vi "CANOpen_Create PDO and Channels.vi"(7 "Type":T1, 8 "error in (no error)":errorcluster, 9 "Cancelled?":bool, 10 "PDO Settings":T3={"Parameters"=[], "PDO Channel"=1, "Start Index"=0, "Length"=0} {"PDO Channel" items=["PDO 1", "PDO 2", "PDO 3", "PDO 4"]; "Parameters"."Bit Offset" max=8 step=1; "Parameters"."Byte Offset" max=8 step=1}, 11 "Item Ref out":T2 format="%.0x") -> (0 "error out":errorcluster, 2 "New PDO":T2=18446744073709551615 format="%.0x")   [LabVIEW 2013]
uses:
  <vilib>/NI Veristand/Custom Device API/Custom Device Item Ref.ctl
  Shared Code/CANOpen_PDO Settings.ctl
  Shared Code/CANOpen_PDO Parameter Settings.ctl
  Shared Code/CANOpen_PDO Data Type.ctl
  CANopen Byte Order.ctl
  CANOpen_PDO Type.ctl
  <vilib>/NI Veristand/Custom Device API/Custom Device Channel.ctl
  <vilib>/NI Veristand/Custom Device API/Custom Device Channel Type.ctl
  Shared Code/CANOpen Addon GUID Lookup Global.vi
  CANOpen Addon Custom Device.lvlib
  <vilib>/NI Veristand/Custom Device API/Custom Device API.lvlib
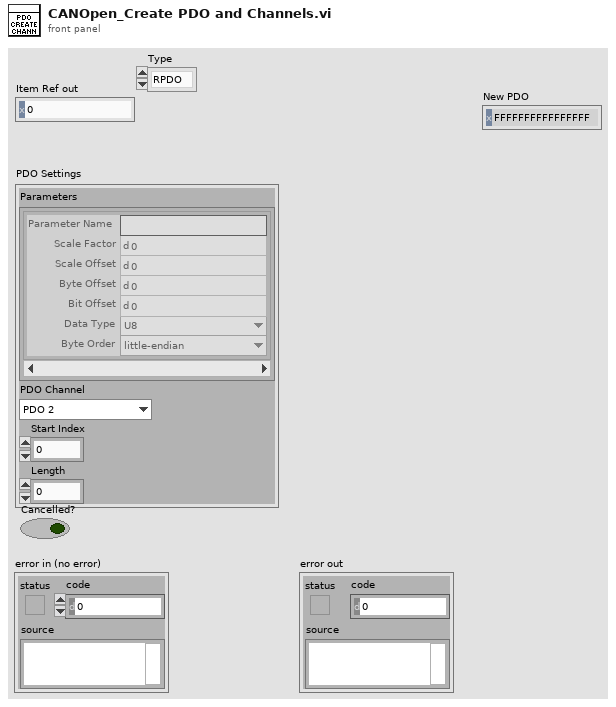
[diagram p1: front panel]
types:
  T1 = typedef "CANOpen_PDO Type.ctl" = enum16{"RPDO", "TPDO"}
  T2 = typedef "Custom Device API.lvlib/Custom Device Item Ref.ctl" = u64
  T3 = typedef "CANOpen Addon Custom Device.lvlib/CANOpen_PDO Settings.ctl" = cluster{"Parameters":T4[], "PDO Channel":u8, "Start Index":u32, "Length":u32}
  T4 = typedef "CANOpen Addon Custom Device.lvlib/CANOpen_PDO Parameter Settings.ctl" = cluster{"Parameter Name":string, "Scale Factor":dbl, "Scale Offset":dbl, "Byte Offset":u8, "Bit Offset":u8, "Data Type":T5, "Byte Order":T6}
  T5 = typedef "CANOpen Addon Custom Device.lvlib/CANOpen_PDO Data Type.ctl" = enum16{"U8", "U16", "U32", "I8", "I16", "I32", "Single", "Double", "Boolean"}
  T6 = typedef "CANOpen Addon Custom Device.lvlib/CANopen Byte Order.ctl" = enum16{"big-endian network order", "little-endian"}
  T7 = typedef "Custom Device API.lvlib/Custom Device Channel.ctl" = cluster{"Type":T8, "Units":string, "Default Value":dbl, "Faultable":bool, "Scalable":bool}
  T8 = typedef "Custom Device API.lvlib/Custom Device Channel Type.ctl" = enum16{"Input", "Output"}
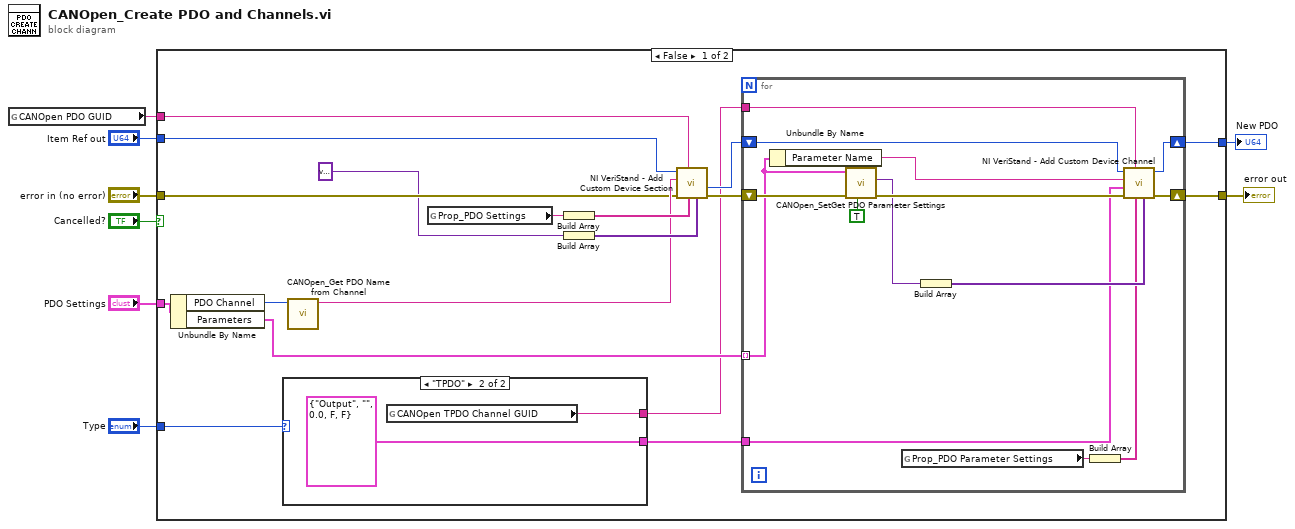
[diagram p0: block diagram]
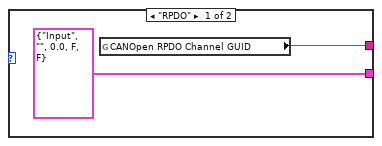
[diagram p2: hidden frame]
diagram:
  n1 = global read "CANOpen Addon GUID Lookup Global.vi" "CANOpen PDO GUID"() -> (w7:string)
  n2 = case shown="False" "Cancelled?" {
    tunnel: w7 -> [w26 _]
    tunnel: [w17 w45] -> w8
    tunnel: "error in (no error)" -> [w11 w45]
    tunnel: "Item Ref out" -> [w25 _]
    tunnel: "PDO Settings" -> [w24 _]
    tunnel: [w14 _] -> w2
    tunnel: "Type" -> [w12 _]
    frame False {
      n3 = Unbundle By Name(w24) -> ("PDO Channel"=w20:u8, "Parameters"=w16:T4[])
      n4 = case shown="\"TPDO\"" w12 {
        tunnel: [T7 {"Type"=enum."Input", "Units"="", "Default Value"=0.0, "Faultable"=FALSE, "Scalable"=FALSE} ("Channel") T7 {"Type"=enum."Output", "Units"="", "Default Value"=0.0, "Faultable"=FALSE, "Scalable"=FALSE} ("Channel")] -> w13
        tunnel: [w27 w29] -> w9
        frame "RPDO" {
          n5 = global read "CANOpen Addon GUID Lookup Global.vi" "CANOpen RPDO Channel GUID"() -> (w27:string)
        }
        frame "TPDO" {
          n6 = global read "CANOpen Addon GUID Lookup Global.vi" "CANOpen TPDO Channel GUID"() -> (w29:string)
        }
      }
      n7 = call "CANOpen_Get PDO Name from Channel.vi"("PDO Channel"=w20) -> ("PDO Channel Name"=w19:string)  [unwired: 10 in]
      n8 = global read "CANOpen Addon GUID Lookup Global.vi" "Prop_PDO Settings"() -> (w23:string)
      n9 = Build Array(w23) -> (w22:string[])
      n10 = Build Array(variant ("variant")) -> (w21:variant[])
      n11 = call <vilib>:"NI VeriStand - Add Custom Device Section.vi"("Property Values"=w21, "Property names"=w22, "GUID (Default Section)"=w26, "error in (no error)"=w11, "Section Name"=w19, "Parent Ref in"=w25) -> ("error out"=w18:errorcluster, "Section Ptr"=w15:T2)  [unwired: 2 in, 2 out]
      n12 = for {
        tunnel: w9 -> [w42]
        shift-right: [w44] -> w17
        shift-left: w18 -> [w41]
        tunnel: w16 -> [w35] mode=indexing
        shift-right: [w32] -> w14
        shift-left: w15 -> [w43]
        tunnel: w13 -> [w31]
        n13 = Unbundle By Name(w35) -> ("Parameter Name"=w34:string)
        n14 = call "CANOpen_SetGet PDO Parameter Settings.vi"("Set Parameters"=TRUE, "error in (no error)"=w41, "PDO Parameter Settings"=w35) -> ("error out"=w37:errorcluster, "Parameters"=w36:variant)  [unwired: 6 in, 1 out]
        n15 = global read "CANOpen Addon GUID Lookup Global.vi" "Prop_PDO Parameter Settings"() -> (w39:string)
        n16 = Build Array(w36) -> (w40:variant[])
        n17 = Build Array(w39) -> (w38:string[])
        n18 = call <vilib>:"NI VeriStand - Add Custom Device Channel.vi"("Property Values"=w40, "Property names"=w38, "GUID (Default Channel)"=w42, "error in (no error)"=w37, "Channel"=w31, "Channel Name"=w34, "Parent Ref in"=w43) -> ("error out"=w44:errorcluster, "Parent Ref out"=w32:T2)  [unwired: 1 in, 2 out]
      }
    }
    frame True {
    }
  }
  "error out" <- w8
  "New PDO" <- w2
